vi "three_button.vi"(7 "callee":refnum<vi>, 8 "error in (no error)":errorcluster, 11 "configuration":T1) -> (0 "error out":errorcluster, 3 "dialog_selection":T2=enum."button_2")   [LabVIEW 2015, in "lv-dialog-interfaces.lvlib"]
uses:
  lv-dialog-interfaces.lvlib
  lv-dialog/api/v1/public/_controls/dialog_selection.ctl
  private/_controls/dialog_type.ctl
  private/_controls/hmi_references.ctl
  private/_controls/configuration.ctl
  <vilib>/event_ctls.llb/eventvkey.ctl
  lv-dialog/api/v1/v1.lvlib
panel:
  out "dialog":string
  in  "button_1":bool
  in  "button_2":bool
  in  "button_3":bool
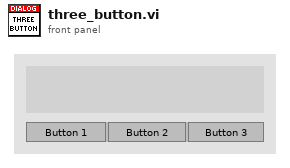
[diagram p1: front panel]
types:
  T1 = cluster{"dialog_text":string, "boolean_text_1":string, "boolean_text_2":string, "boolean_text_3":string}
  T2 = typedef "lv-dialog.lvlib/v1.lvlib/dialog_selection.ctl" = enum16{"null", "panel_closed", "button_1", "button_2", "button_3", "cancelled"}
  T3 = typedef "lv-dialog-interfaces.lvlib/dialog_type.ctl" = enum16{"null", "one_button", "two_button", "three_button", "confirmation", "busy_wait", "error", "busy_wait_embed", "combo_box", "data_entry_string", "data_entry_numeric"}
  T4 = typedef "lv-dialog-interfaces.lvlib/configuration.ctl" = cluster{"dialog_text":string, "boolean_text_1":string, "boolean_text_2":string, "boolean_text_3":string, "inner_color":u32, "outer_color":u32, "wait_s":dbl, "error_status":bool, "error_source":string, "error_details":string, "string []":string[], "custom_entry":bool}
  T5 = typedef "lv-dialog-interfaces.lvlib/hmi_references.ctl" = cluster{"vi_reference":refnum<vi>, "caller":refnum<vi>, "dialog":refnum<vi>, "button_1":refnum<vi>, "button_2":refnum<vi>, "button_3":refnum<vi>, "busy":refnum<vi>, "error_glyph":refnum<vi>, "error_source":refnum<vi>, "error_text":refnum<vi>, "combo_box":refnum<vi>}
  T6 = typedef "eventvkey.ctl" = enum16{"ASCII", "Enter", "Return", "Shift", "Ctrl", "Alt", "Cmd", "Opt", "Caps", "NumLock", "Clear", "Break", "Up", "Down", "Left", "Right", "Insert", "Delete", "Home", "End", "PageUp", "PageDown", "Escape", "Help", "Pause", "ScrollLock", "F1", "F2", "F3", "F4", "F5", "F6", "F7", "F8", "F9", "F10", "F11", "F12", "F13", "F14", "F15", "F16", "F17", "F18", "F19", "F20", "F21", "F22", "F23", "F24", "Play", "VolumeUp", "VolumeDown", "Mute", "Two Byte Char"}
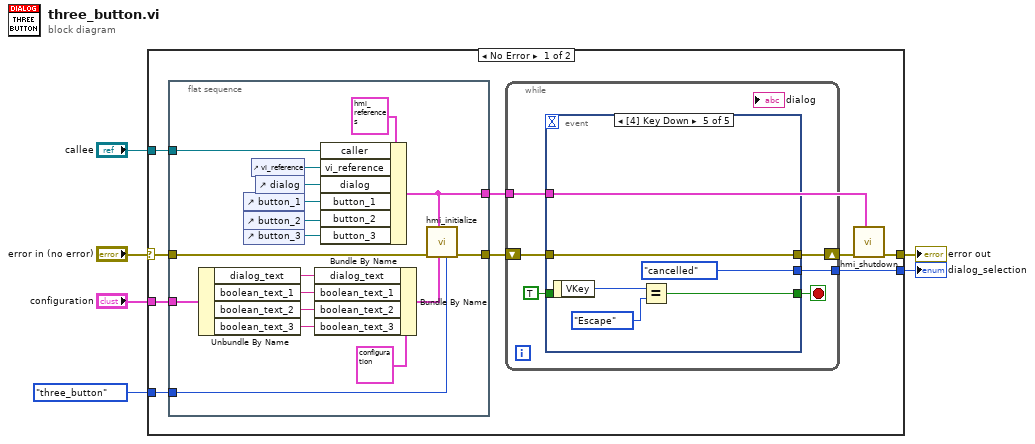
[diagram p0: block diagram]
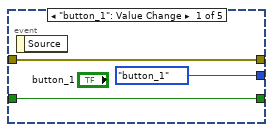
[diagram p2: hidden frame]
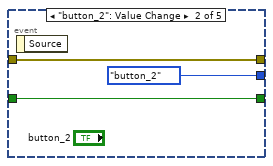
[diagram p3: hidden frame]
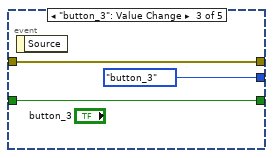
[diagram p4: hidden frame]
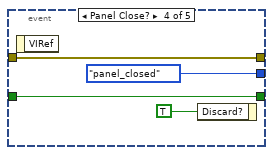
[diagram p5: hidden frame]
diagram:
  n1 = case shown="No Error" "error in (no error)" {
    selector: "error in (no error)" -> [w15 w58]
    tunnel: dialog_type."three_button" ("dialog_type") -> [w14 _]
    tunnel: [w12 _] -> w2
    tunnel: "callee" -> [w11 _]
    tunnel: [w9 w58] -> w3
    tunnel: "configuration" -> [w8 _]
    frame No Error {
      n2 = flat-sequence {
        tunnel: w15 -> [w25]
        tunnel: w14 -> [w29]
        tunnel: [w28] -> w13
        tunnel: w11 -> [w24]
        tunnel: [w23] -> w7
        tunnel: w8 -> [w22]
        frame #0 {
          n3 = Unbundle By Name(w22) -> ("dialog_text"=w20:string, "boolean_text_1"=w18:string, "boolean_text_2"=w17:string, "boolean_text_3"=w16:string)
          n4 = control-ref of="button_1"() -> (w31:refnum<vi>)
          n5 = control-ref of="button_2"() -> (w27:refnum<vi>)
          n6 = control-ref of="button_3"() -> (w26:refnum<vi>)
          n7 = control-ref of="vi_reference"() -> (w33:refnum<vi>)
          n8 = control-ref of="dialog"() -> (w32:refnum<vi>)
          n9 = Bundle By Name(cluster=T4 {"dialog_text"="", "boolean_text_1"="", "boolean_text_2"="", "boolean_text_3"="", "inner_color"=16711680, "outer_color"=6618880, "wait_s"=nan, "error_status"=FALSE, "error_source"="", "error_details"="", "string []"=[], "custom_entry"=FALSE} ("configuration"), "dialog_text"=w20, "boolean_text_1"=w18, "boolean_text_2"=w17, "boolean_text_3"=w16) -> (w19:T4)
          n10 = Bundle By Name(cluster=T5 {"vi_reference"=refnum, "caller"=refnum, "dialog"=refnum, "button_1"=refnum, "button_2"=refnum, "button_3"=refnum, "busy"=refnum, "error_glyph"=refnum, "error_source"=refnum, "error_text"=refnum, "combo_box"=refnum}, "caller"=w24, "vi_reference"=w33, "dialog"=w32, "button_1"=w31, "button_2"=w27, "button_3"=w26) -> (w23:T5)
          n11 = call "hmi_initialize.vi"("dialog_type"=w29, "configuration"=w19, "references"=w23, "error in (no error)"=w25) -> ("error out"=w28:errorcluster)  [unwired: 7 in]
        }
      }
      n12 = while {
        tunnel: [w38] -> w12
        shift-right: [w36] -> w10
        shift-left: w13 -> [w39]
        tunnel: w7 -> [w37]
        stop <- w34 stop-if-true
        n13 = event shown="[4] Key Down" {
          selector: _ -> [_ _ _ _ _]
          dyn-events: _ -> [_ _ _ _ _]
          timeout: _ -> [_ _ _ _ _]
          tunnel: w39 -> [w42 w45 w48 w51 w57]
          tunnel: [w42 w45 w48 w51 w57] -> w36
          tunnel: [dialog_selection."button_1" ("dialog_selection") dialog_selection."button_2" ("dialog_selection") dialog_selection."button_3" ("dialog_selection") dialog_selection."panel_closed" ("dialog_selection") dialog_selection."cancelled" ("dialog_selection")] -> w38
          tunnel: w37 -> [_ _ _ _ _]
          tunnel: [w40 w43 w46 w49 w53] -> w34
          tunnel: TRUE -> [w40 w43 w46 w49 _]
          event "button_1": Value Change {
            n14 = event-data() -> ()  [unwired: 1 in, 1 out]
          }
          event "button_2": Value Change {
            n15 = event-data() -> ()  [unwired: 1 in, 1 out]
          }
          event "button_3": Value Change {
            n16 = event-data() -> ()  [unwired: 1 in, 1 out]
          }
          event Panel Close? {
            n17 = event-data() -> ()  [unwired: 1 in, 1 out]
            n18 = event-data("Discard?"=TRUE) -> ()  [unwired: 1 in, 1 out]
          }
          event Key Down {
            n19 = event-data() -> ("VKey"=w55:T6)  [unwired: 1 in]
            n20 = Equal?(x=w55, y=eventvkey."Escape" ("VKey")) -> (x = y?=w53:bool)
          }
        }
      }
      n21 = call "hmi_shutdown.vi"("references"=w7, "error in (no error)"=w10) -> ("error out"=w9:errorcluster)  [unwired: 9 in]
    }
    frame Error {
    }
  }
  "error out" <- w3
  "dialog_selection" <- w2
